vi "close.vi"(8 "error in (no error)":errorcluster, 11 "TCPConnection In":refnum<class "TCPConnection.lvclass">) -> (0 "error out":errorcluster, 3 "TCPConnection Out":refnum<class "TCPConnection.lvclass">)   [LabVIEW 2023, in "AbstractFactory.lvlib" / "TCPConnection.lvclass"]
uses:
  TCPConnection.lvclass
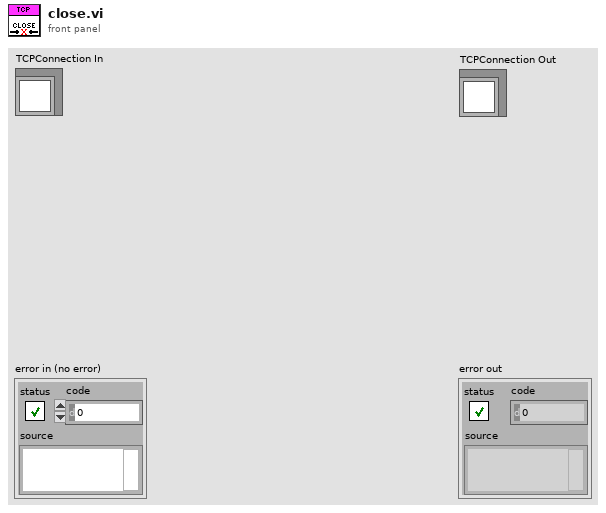
[diagram p1: front panel]
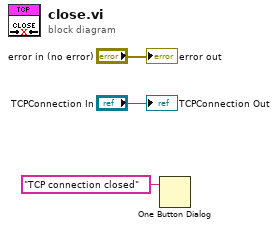
[diagram p0: block diagram]
diagram:
  n1 = One Button Dialog(message="TCP connection closed") -> ()  [unwired: 1 in, 1 out]
  "error out" <- "error in (no error)"
  "TCPConnection Out" <- "TCPConnection In"
